vi "MKS670_Status.vi"() -> (1 "n_ng":u8, 2 "values":T1)   [LabVIEW 2019]
uses:
  MKS670_Global.vi
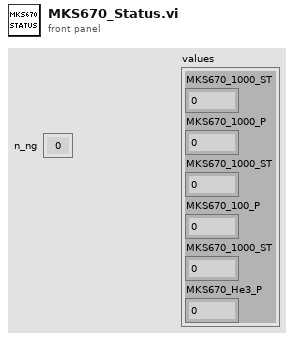
[diagram p1: front panel]
types:
  T1 = cluster{"MKS670_1000_ST":u32, "MKS670_1000_P":dbl, "MKS670_1000_ST":u32, "MKS670_100_P":dbl, "MKS670_1000_ST":u32, "MKS670_He3_P":dbl}
  T2 = enum32{"Bad", "Idle", "Run top level", "Running"}
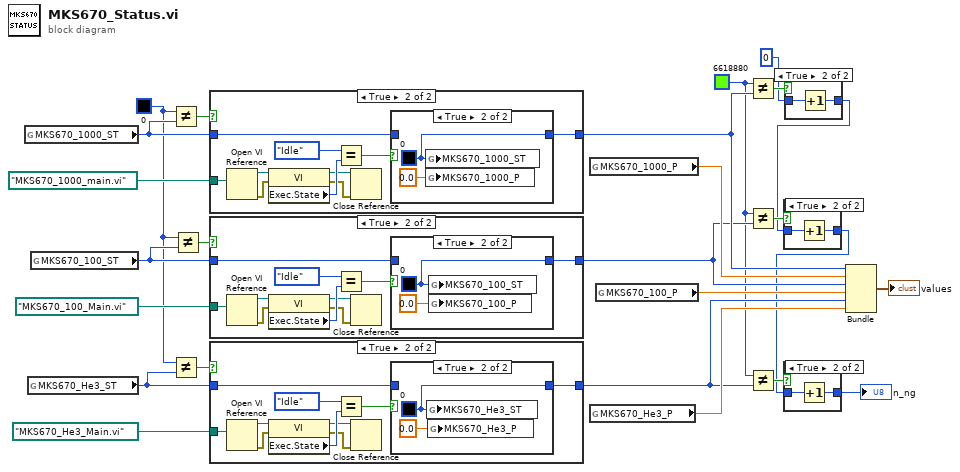
[diagram p0: block diagram]
diagram:
  w8 = u32 6618880 ("MKS670_1000_ST 2")
  w17 = u32 0 ("MKS670_1000_ST 2")
  n1 = global read "MKS670_Global.vi" "MKS670_1000_ST"() -> (w24:u32)
  n2 = global read "MKS670_Global.vi" "MKS670_He3_ST"() -> (w16:u32)
  n3 = global read "MKS670_Global.vi" "MKS670_100_ST"() -> (w20:u32)
  n4 = Not Equal?(x=w17, y=w24) -> (x != y?=w25:bool)
  n5 = Not Equal?(x=w17, y=w16) -> (x != y?=w18:bool)
  n6 = Not Equal?(x=w17, y=w20) -> (x != y?=w21:bool)
  n7 = case shown="True" w25 {
    tunnel: w24 -> [w26 w28]
    tunnel: [w26 w27] -> w11
    tunnel: path "MKS670_1000_main.vi" ("vi path") -> [_ w29]
    frame False {
    }
    frame True {
      n8 = Open VI Reference(vi path=w29) -> (vi reference=w36:refnum<vi>, error out=w35:errorcluster)  [unwired: 5 in]
      n9 = property class="VI"(reference=w36, error in=w35) -> (reference out=w31:refnum<vi>, error out=w30:errorcluster, "Exec.State"=w33:T2)
      n10 = Equal?(x=T2."Idle" ("Execution:State"), y=w33) -> (x = y?=w34:bool)
      n11 = Close Reference(reference=w31, error in (no error)=w30) -> ()  [unwired: 1 out]
      n12 = case shown="True" w34 {
        tunnel: w28 -> [w37 _]
        tunnel: [w37 w38] -> w27
        frame False {
        }
        frame True {
          w38 = u32 0 ("MKS670_1000_ST")
          n13 = global write "MKS670_Global.vi" "MKS670_1000_ST"(w38) -> ()
          n14 = global write "MKS670_Global.vi" "MKS670_1000_P"(0.0 ("MKS670_1000_P")) -> ()
        }
      }
    }
  }
  n15 = case shown="True" w21 {
    tunnel: w20 -> [w40 w42]
    tunnel: [w40 w41] -> w10
    tunnel: path "MKS670_100_Main.vi" ("vi path") -> [_ w43]
    frame False {
    }
    frame True {
      n16 = Open VI Reference(vi path=w43) -> (vi reference=w50:refnum<vi>, error out=w49:errorcluster)  [unwired: 5 in]
      n17 = property class="VI"(reference=w50, error in=w49) -> (reference out=w45:refnum<vi>, error out=w44:errorcluster, "Exec.State"=w47:T2)
      n18 = Equal?(x=T2."Idle" ("Execution:State"), y=w47) -> (x = y?=w48:bool)
      n19 = Close Reference(reference=w45, error in (no error)=w44) -> ()  [unwired: 1 out]
      n20 = case shown="True" w48 {
        tunnel: w42 -> [w51 _]
        tunnel: [w51 w52] -> w41
        frame False {
        }
        frame True {
          w52 = u32 0 ("MKS670_1000_ST")
          n21 = global write "MKS670_Global.vi" "MKS670_100_ST"(w52) -> ()
          n22 = global write "MKS670_Global.vi" "MKS670_100_P"(0.0 ("MKS670_1000_P")) -> ()
        }
      }
    }
  }
  n23 = case shown="True" w18 {
    tunnel: w16 -> [w54 w56]
    tunnel: [w54 w55] -> w9
    tunnel: path "MKS670_He3_Main.vi" ("vi path") -> [_ w57]
    frame False {
    }
    frame True {
      n24 = Open VI Reference(vi path=w57) -> (vi reference=w64:refnum<vi>, error out=w63:errorcluster)  [unwired: 5 in]
      n25 = property class="VI"(reference=w64, error in=w63) -> (reference out=w59:refnum<vi>, error out=w58:errorcluster, "Exec.State"=w61:T2)
      n26 = Equal?(x=T2."Idle" ("Execution:State"), y=w61) -> (x = y?=w62:bool)
      n27 = Close Reference(reference=w59, error in (no error)=w58) -> ()  [unwired: 1 out]
      n28 = case shown="True" w62 {
        tunnel: w56 -> [w65 _]
        tunnel: [w65 w66] -> w55
        frame False {
        }
        frame True {
          w66 = u32 0 ("MKS670_1000_ST")
          n29 = global write "MKS670_Global.vi" "MKS670_He3_ST"(w66) -> ()
          n30 = global write "MKS670_Global.vi" "MKS670_He3_P"(0.0 ("MKS670_1000_P")) -> ()
        }
      }
    }
  }
  n31 = global read "MKS670_Global.vi" "MKS670_1000_P"() -> (w22:dbl)
  n32 = global read "MKS670_Global.vi" "MKS670_He3_P"() -> (w13:dbl)
  n33 = global read "MKS670_Global.vi" "MKS670_100_P"() -> (w14:dbl)
  n34 = Not Equal?(x=w8, y=w11) -> (x != y?=w7:bool)
  n35 = Not Equal?(x=w8, y=w10) -> (x != y?=w5:bool)
  n36 = Not Equal?(x=w8, y=w9) -> (x != y?=w3:bool)
  n37 = case shown="True" w7 {
    tunnel: u8 0 ("n_idle") -> [w68 w70]
    tunnel: [w68 w69] -> w4
    frame False {
    }
    frame True {
      n38 = Increment(x=w70) -> (x+1=w69:u8)
    }
  }
  n39 = case shown="True" w5 {
    tunnel: w4 -> [w71 w73]
    tunnel: [w71 w72] -> w2
    frame False {
    }
    frame True {
      n40 = Increment(x=w73) -> (x+1=w72:u8)
    }
  }
  n41 = case shown="True" w3 {
    tunnel: w2 -> [w74 w76]
    tunnel: [w74 w75] -> w1
    frame False {
    }
    frame True {
      n42 = Increment(x=w76) -> (x+1=w75:u8)
    }
  }
  "n_ng" <- w1
  n43 = Bundle("MKS670_1000_ST"=w11, "MKS670_1000_P"=w22, "MKS670_1000_ST"=w10, "MKS670_100_P"=w14, "MKS670_1000_ST"=w9, "MKS670_He3_P"=w13) -> (→"values":T1)  [unwired: 1 in]
